vi "Write sessions.vi"(8 "error in (no error)":errorcluster, 10 "sessions":refnum<k20>[](array[refnum]), 11 "NIScope in":refnum<class "NIScope.lvclass">) -> (0 "error out":errorcluster, 3 "NIScope out":refnum<class "NIScope.lvclass">)   [LabVIEW 2014, in "ScopePlugins.lvlib" / "NIScope.lvclass"]
uses:
  NIScope.lvclass
  NIScope.lvclass/NIScope.ctl
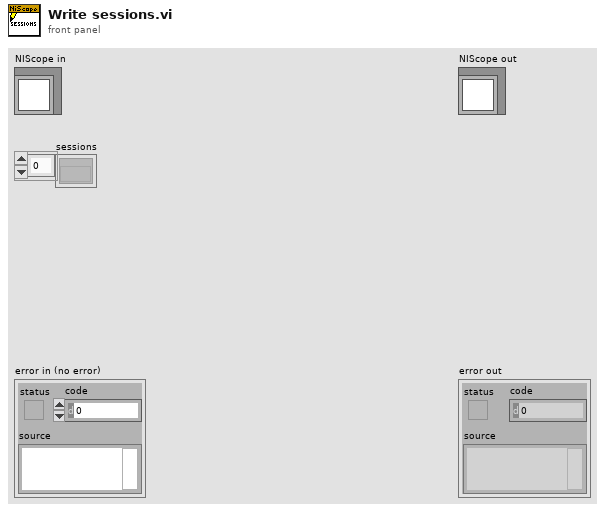
[diagram p1: front panel]
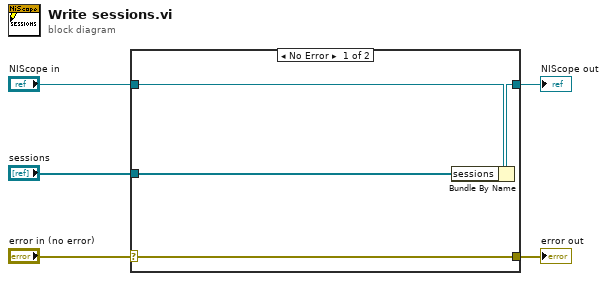
[diagram p0: block diagram]
diagram:
  n1 = case shown="No Error" "error in (no error)" {
    selector: "error in (no error)" -> [w9 w10]
    tunnel: [w9 w10] -> w4
    tunnel: [w7 w11] -> w2
    tunnel: "NIScope in" -> [w8 w11]
    tunnel: "sessions" -> [w6 _]
    frame No Error {
      n2 = Bundle By Name(cluster=w8, "sessions"=w6) -> (w7:refnum<class "NIScope.lvclass">)
    }
    frame Error {
    }
  }
  "error out" <- w4
  "NIScope out" <- w2
